vi "Enable Measurement Auto Range.vi"(8 "error in (no error)":errorcluster, 9 "Enable Auto Range (T:Enable)":bool=TRUE, 10 "Function (0: Volts)":u16(ring) items=["Volts", "Current", "Resistance"], 11 "VISA resource name":refnum<visa-resource-name>) -> (0 "error out":errorcluster, 3 "VISA resource name out":refnum<visa-resource-name>)   [LabVIEW 2022 SP3, in "Keithley 2450.lvlib"]
doc: "Configures the measurement auto range on the instrument."
uses:
  Keithley 2450.lvlib
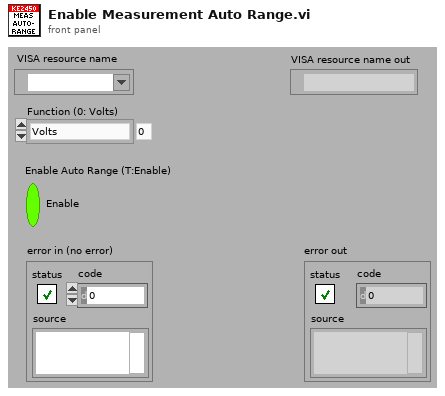
[diagram p1: front panel]
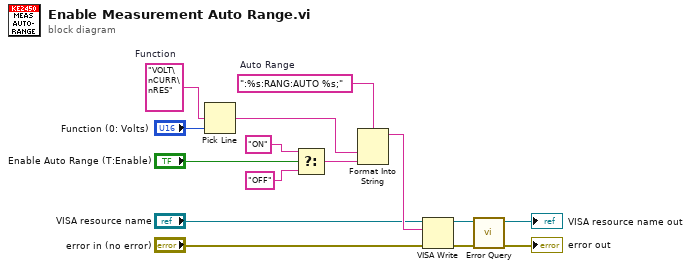
[diagram p0: block diagram]
diagram:
  w5 = "VOLT\nCURR\nRES"  # Function
  w11 = ":%s:RANG:AUTO %s;"  # Auto Range
  n1 = Pick Line(multi-line string=w5, line index="Function (0: Volts)") -> (output string=w3:string)  [unwired: 1 out]
  n2 = Select(t="ON", s="Enable Auto Range (T:Enable)", f="OFF") -> (s? t:f=w8:string)
  n3 = Format Into String(format string=w11, w3, w8) -> (resulting string=w7:string)  [unwired: 2 in, 1 out]
  n4 = VISA Write(VISA resource name="VISA resource name", write buffer=w7, error in (no error)="error in (no error)") -> (VISA resource name out=w13:refnum<visa-resource-name>, error out=w12:errorcluster)  [unwired: 1 out]
  n5 = call "Error Query.vi"("error in (no error)"=w12, "VISA resource name"=w13) -> ("error out"=→"error out":errorcluster, "VISA resource name out"=→"VISA resource name out":refnum<visa-resource-name>)  [unwired: 8 out]
